vi "Main.vi"(8 "error in (no error)":errorcluster) -> (0 "error out":errorcluster)   [LabVIEW 2015]
uses:
  Parse Presentation/Parse Presentation.lvclass
panel:
  out "Output Directory":path
  in  "PPT Path":path
  # "D:\\Metis Automation\\Test Import.pptx"
  # "D:\\Metis Automation\\Tactus.pptx"
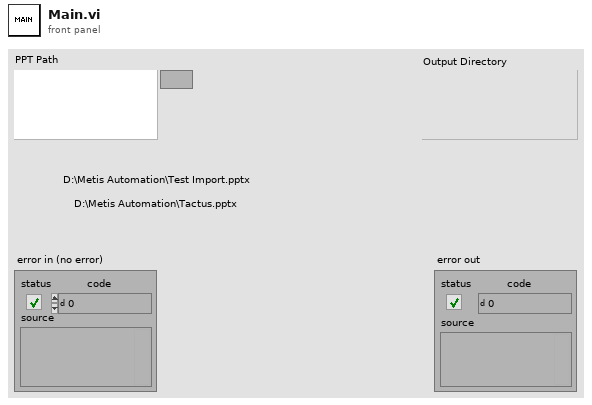
[diagram p1: front panel]
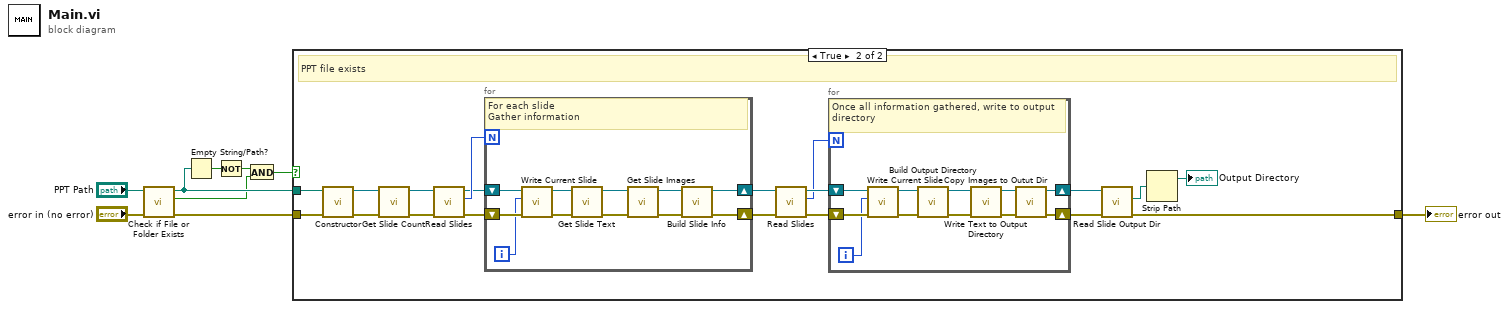
[diagram p0: block diagram]
diagram:
  n1 = call <vilib>:"Check if File or Folder Exists.vi"("error in (no error)"="error in (no error)", "path"="PPT Path") -> ("error out"=w7:errorcluster, "file or folder exists?"=w2:bool, "dup path"=w5:path)  [unwired: 7 in]
  n2 = Empty String/Path?(string/path=w5) -> (empty?=w4:bool)
  n3 = Not(x=w4) -> (.not. x?=w3:bool)
  n4 = And(x=w3, y=w2) -> (x .and. y?=w1:bool)
  n5 = case shown="True" w1 {
    tunnel: [w10 w14] -> w8
    tunnel: w7 -> [w10 w29]
    tunnel: w5 -> [_ w28]
    frame False {
    }
    frame True {
      # "PPT file exists"
      n6 = call "Constructor.vi"("error in (no error)"=w29, "PPT Path"=w28) -> ("error out"=w27:errorcluster, "Parse Presentation out"=w26:refnum<class "Parse Presentation.lvclass">)  [unwired: 8 in]
      n7 = call "Get Slide Count.vi"("error in (no error)"=w27, "Parse Presentation in"=w26) -> ("error out"=w24:errorcluster, "Parse Presentation out"=w25:refnum<class "Parse Presentation.lvclass">)  [unwired: 8 in]
      n8 = call-dynamic "Read Slides.vi"("error in (no error)"=w24, "Parse Presentation in"=w25) -> ("error out"=w23:errorcluster, "Slides"=w22:i32, "Parse Presentation out"=w21:refnum<class "Parse Presentation.lvclass">)  [unwired: 7 in]
      n9 = for {
        N: w22 -> [_]
        shift-right: [w41] -> w20
        shift-left: w23 -> [w51]
        shift-right: [w43] -> w18
        shift-left: w21 -> [w50]
        i -> [w49]
        # "For each slide\nGather information"
        n10 = call-dynamic "Write Current Slide.vi"("error in (no error)"=w51, "Current Slide"=w49, "Parse Presentation in"=w50) -> ("error out"=w47:errorcluster, "Parse Presentation out"=w48:refnum<class "Parse Presentation.lvclass">)  [unwired: 7 in]
        n11 = call "Get Slide Text.vi"("error in (no error)"=w47, "Parse Presentation in"=w48) -> ("error out"=w45:errorcluster, "Parse Presentation out"=w46:refnum<class "Parse Presentation.lvclass">)  [unwired: 8 in]
        n12 = call "Get Slide Images.vi"("error in (no error)"=w45, "Parse Presentation in"=w46) -> ("error out"=w42:errorcluster, "Parse Presentation out"=w44:refnum<class "Parse Presentation.lvclass">)  [unwired: 8 in]
        n13 = call "Build Slide Info.vi"("error in (no error)"=w42, "Parse Presentation in"=w44) -> ("error out"=w41:errorcluster, "Parse Presentation out"=w43:refnum<class "Parse Presentation.lvclass">)  [unwired: 8 in]
      }
      n14 = call-dynamic "Read Slides.vi"("error in (no error)"=w20, "Parse Presentation in"=w18) -> ("error out"=w19:errorcluster, "Slides"=w16:i32, "Parse Presentation out"=w17:refnum<class "Parse Presentation.lvclass">)  [unwired: 7 in]
      n15 = for {
        N: w16 -> [_]
        shift-right: [w31] -> w13
        shift-left: w17 -> [w40]
        shift-right: [w30] -> w15
        shift-left: w19 -> [w39]
        i -> [w38]
        # "Once all information gathered, write to output directory"
        n16 = call-dynamic "Write Current Slide.vi"("error in (no error)"=w39, "Current Slide"=w38, "Parse Presentation in"=w40) -> ("error out"=w37:errorcluster, "Parse Presentation out"=w36:refnum<class "Parse Presentation.lvclass">)  [unwired: 7 in]
        n17 = call "Build Output Directory.vi"("error in (no error)"=w37, "Parse Presentation in"=w36) -> ("error out"=w35:errorcluster, "Parse Presentation out"=w34:refnum<class "Parse Presentation.lvclass">)  [unwired: 8 in]
        n18 = call "Write Text to Output Directory.vi"("error in (no error)"=w35, "Parse Presentation in"=w34) -> ("error out"=w32:errorcluster, "Parse Presentation out"=w33:refnum<class "Parse Presentation.lvclass">)  [unwired: 8 in]
        n19 = call "Copy Images to Outut Dir.vi"("error in (no error)"=w32, "Parse Presentation in"=w33) -> ("error out"=w30:errorcluster, "Parse Presentation out"=w31:refnum<class "Parse Presentation.lvclass">)  [unwired: 8 in]
      }
      n20 = call-dynamic "Read Slide Output Dir.vi"("error in (no error)"=w15, "Parse Presentation in"=w13) -> ("error out"=w14:errorcluster, "Slide Output Dir"=w12:path)  [unwired: 7 in, 1 out]
      n21 = Strip Path(path=w12) -> (stripped path=→"Output Directory":path)  [unwired: 1 out]
    }
  }
  "error out" <- w8
